vi "front_panel.vi"() -> ()   [LabVIEW 2020]
uses:
  kontolka.ctl
panel:
  out "unsigned 32bit integer":u32
  in  "Tab Control":enum32{"Page 1", "Page 2"}(tab)
  in  "Record Button":bool
  in  "Play Button":bool
  in  "Media Stop Button":bool
  out "Output panel":T1
  in  "Stop Button":bool
  in  "Control panel":T2
  in  "Open Button":bool
  in  "Save Button":bool
  in  "Configuration name":string
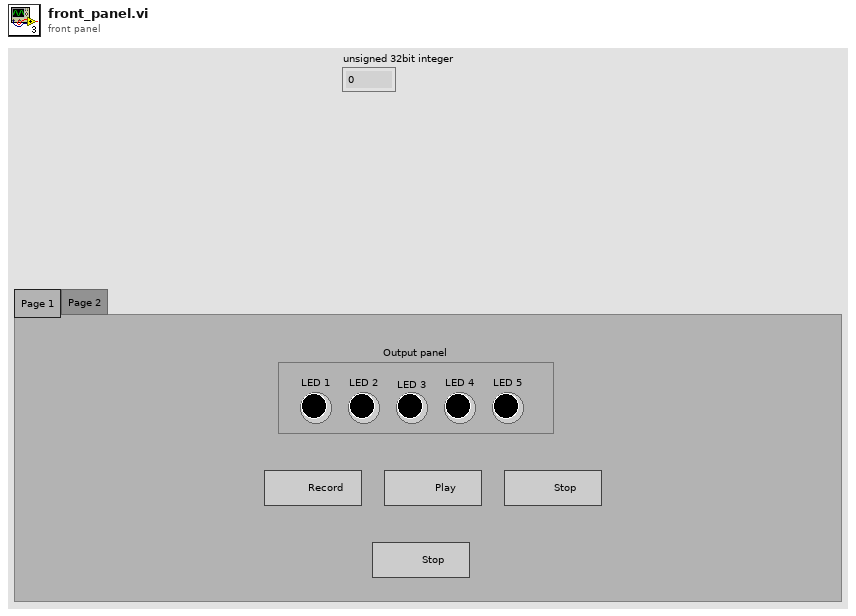
[diagram p1: front panel]
types:
  T1 = cluster{"LED 1":bool, "LED 2":bool, "LED 3":bool, "LED 4":bool, "LED 5":bool}
  T2 = cluster{"  LED 1":cluster{"Wait time":dbl, "Duration time":dbl, "Color":u32}, "  LED 2":cluster{"Wait time":dbl, "Duration time":dbl, "Color":u32}, "LED 3":cluster{"Wait time":dbl, "Duration time":dbl, "Color":u32}, "LED 4":cluster{"Wait time":dbl, "Duration time":dbl, "Color":u32}, " LED 5":cluster{"Wait time":dbl, "Duration time":dbl, "Color":u32}}
  T3 = typedef "kontolka.ctl" = enum16{"Init", "Record", "Play", "Stop", "Open", "Save", "PreparePlay"}
  T4 = enum32{"Page Enabled", "Page Disabled", "Page Disabled & Grayed"}
  T5 = cluster{"Wait time":dbl, "Duration time":dbl, u32}
  T6 = enum8{"Enabled", "Disabled", "Disabled and Grayed Out"}
  T7 = cluster{cluster{"String":i32, "String":i32, "String":i32}, cluster{"String":i32, "String":i32, "String":i32}, cluster{"String":i32, "String":i32, "String":i32}, cluster{"String":i32, "String":i32, "String":i32}, cluster{"String":i32, "String":i32, "String":i32}}
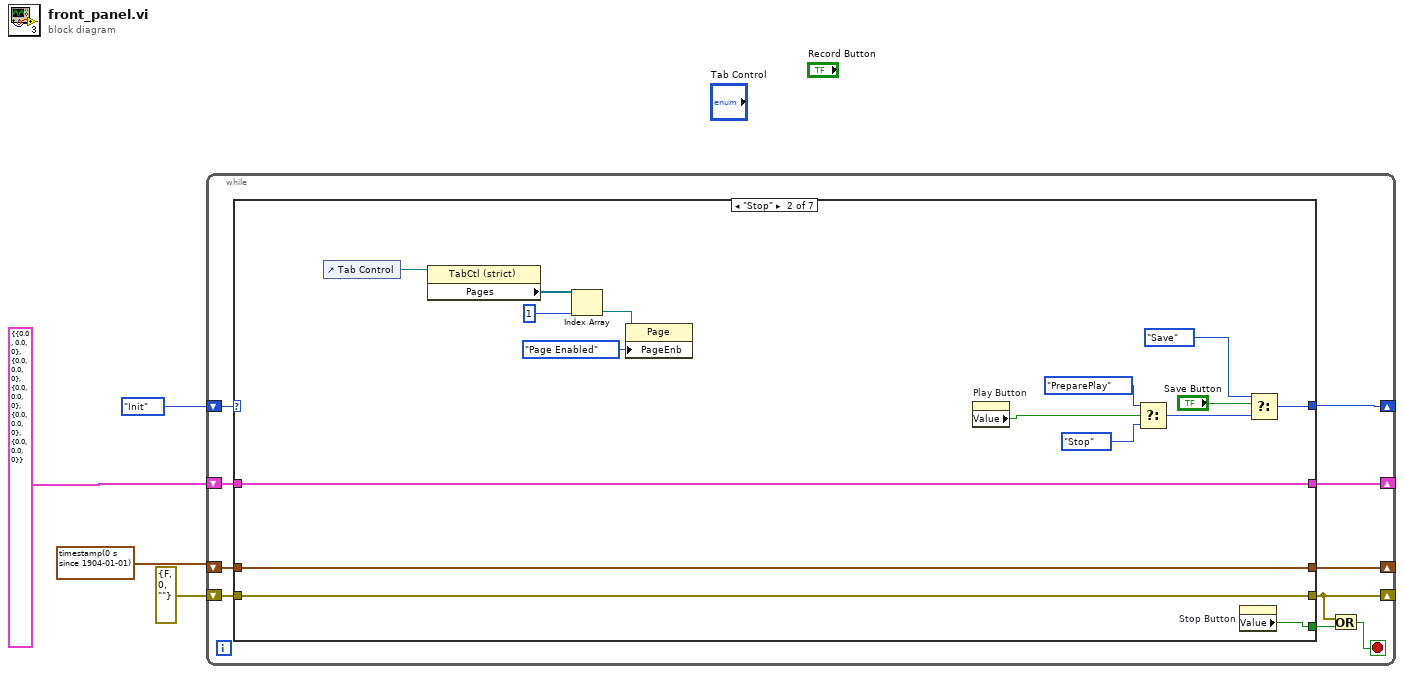
[diagram p0: block diagram]
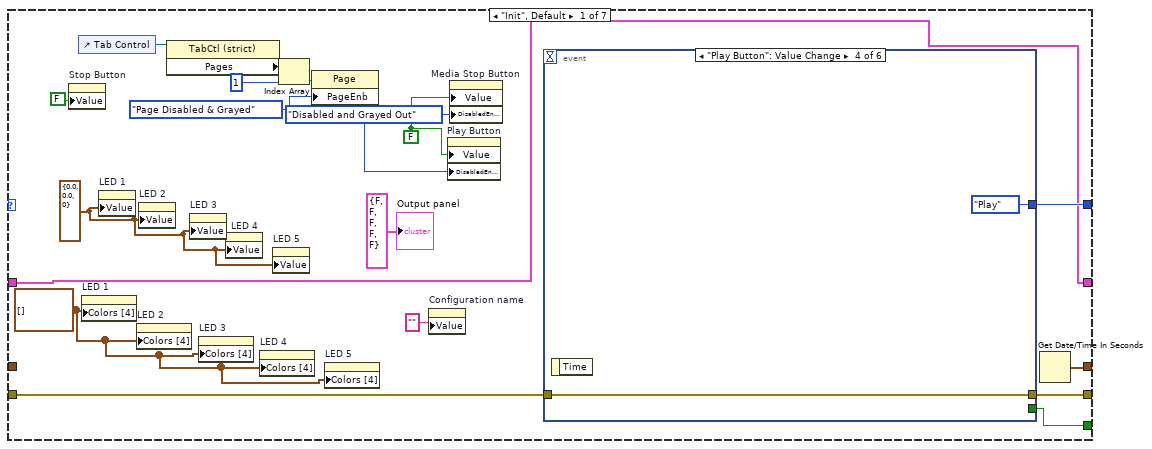
[diagram p2: hidden frame]
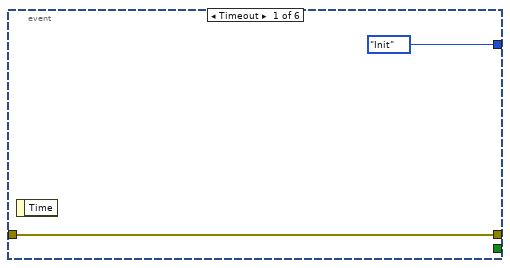
[diagram p3: hidden frame]
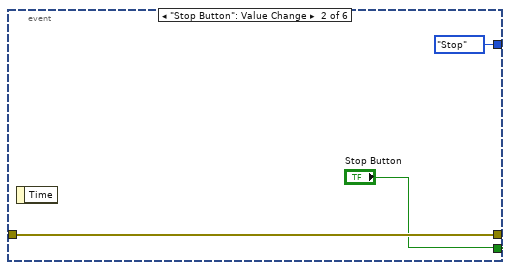
[diagram p4: hidden frame]
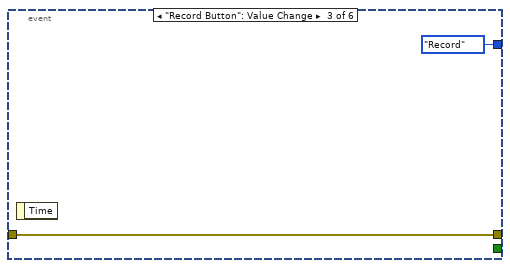
[diagram p5: hidden frame]
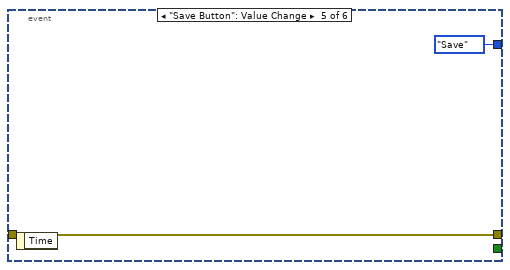
[diagram p6: hidden frame]
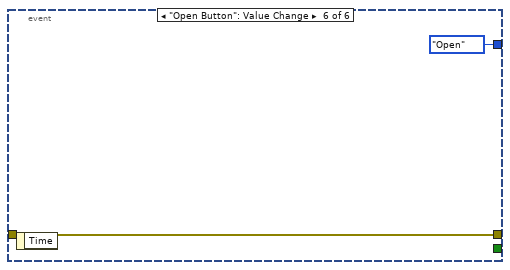
[diagram p7: hidden frame]
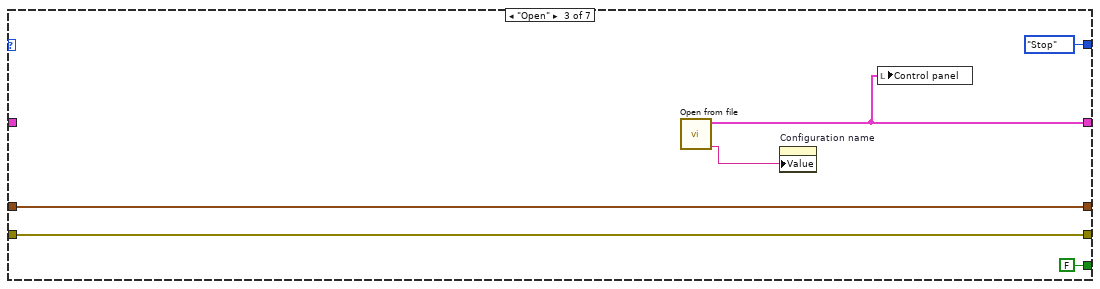
[diagram p8: hidden frame]
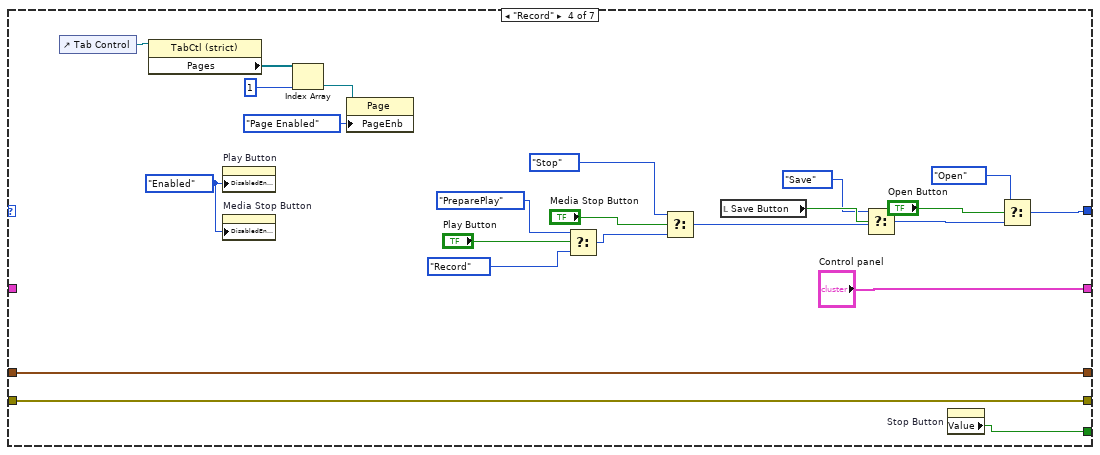
[diagram p9: hidden frame]
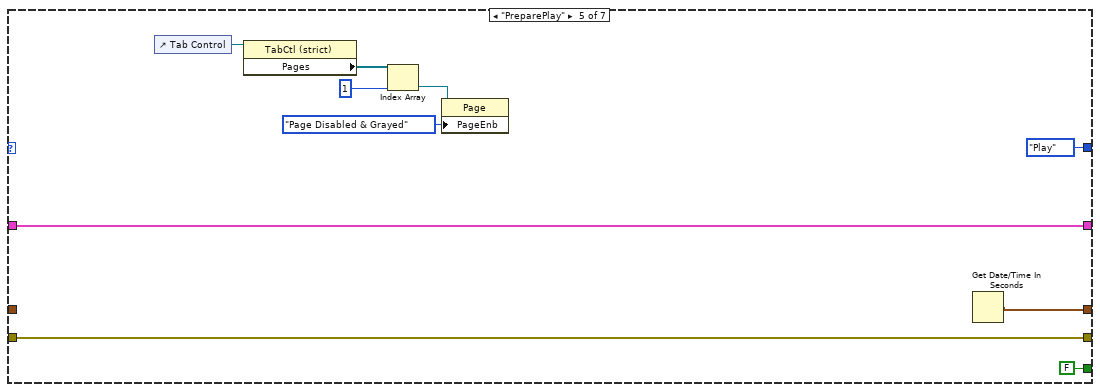
[diagram p10: hidden frame]
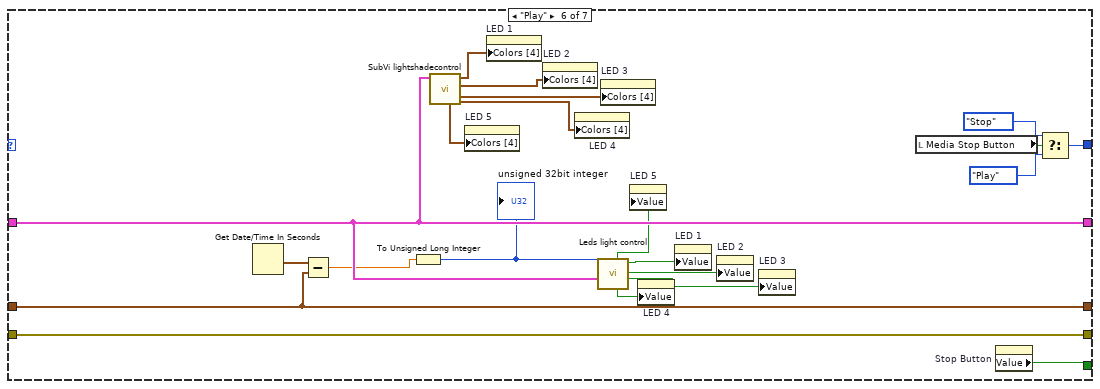
[diagram p11: hidden frame]
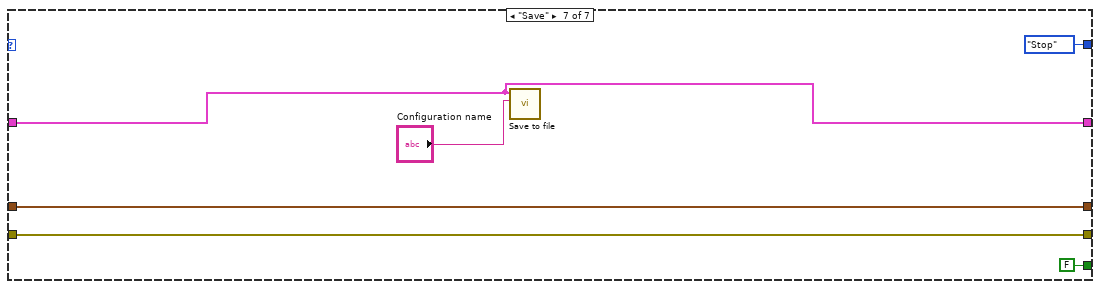
[diagram p12: hidden frame]
diagram:
  n1 = while {
    shift-right: [w11] -> _
    shift-left: errorcluster {"status"=FALSE, "code"=0, "source"=""} ("error constant") -> [w14]
    shift-right: [w5] -> _
    shift-left: kontolka."Init" ("Enum") -> [w10]
    shift-right: [w9] -> _
    shift-left: timestamp(0 s since 1904-01-01) ("seconds since 1Jan1904") -> [w8]
    shift-right: [w7] -> _
    shift-left: T2 {"  LED 1"={"Wait time"=0.0, "Duration time"=0.0, "Color"=0}, "  LED 2"={"Wait time"=0.0, "Duration time"=0.0, "Color"=0}, "LED 3"={"Wait time"=0.0, "Duration time"=0.0, "Color"=0}, "LED 4"={"Wait time"=0.0, "Duration time"=0.0, "Color"=0}, " LED 5"={"Wait time"=0.0, "Duration time"=0.0, "Color"=0}} ("Control panel") -> [w6]
    stop <- w12 stop-if-true
    n2 = case shown="\"Stop\"" w10 {
      tunnel: [w30 w60 w65 w90 w99 w121 w123] -> w11
      tunnel: w14 -> [w31 w60 w65 w90 w99 w121 w123]
      tunnel: [w29 w61 FALSE ("Value") w79 FALSE ("Value") w120 FALSE ("Value")] -> w13
      tunnel: [w32 w46 kontolka."Stop" ("Enum") w72 kontolka."Play" ("Enum") w119 kontolka."Stop" ("Enum")] -> w5
      tunnel: [w23 w59 w66 w78 w98 w108 w124] -> w9
      tunnel: w8 -> [_ w59 w66 w78 _ w108 w124]
      tunnel: [w21 w58 w62 "Control panel" w97 w110 w126] -> w7
      tunnel: w6 -> [w21 w58 _ _ w97 w110 w126]
      frame "Init", Default {
        w15 = cluster{u32, u32}[] [] ("Colors [4]")
        w17 = T5 {"Wait time"=0.0, "Duration time"=0.0, 0} ("Value")
        w19 = T6."Disabled and Grayed Out" ("Disabled")
        w20 = FALSE ("Media Stop Button")
        n3 = property on="Stop Button" class="Bool (strict)"("Value"=FALSE ("Stop Button")) -> ()  [unwired: 2 in, 2 out]
        n4 = control-ref of="Tab Control"() -> (w24:refnum<vi>)
        n5 = property on="LED 1" class="Bool (strict)"("Colors [4]"=w15) -> ()  [unwired: 2 in, 2 out]
        n6 = property on="LED 1" class="Clust (strict)"("Value"=w17) -> ()  [unwired: 2 in, 2 out]
        n7 = property on="LED 2" class="Bool (strict)"("Colors [4]"=w15) -> ()  [unwired: 2 in, 2 out]
        n8 = property on="LED 2" class="Clust (strict)"("Value"=w17) -> ()  [unwired: 2 in, 2 out]
        n9 = property on="Property Node" class="TabCtl (strict)"(reference=w24) -> ("Pages"=w27:refnum<vi>[])  [unwired: 1 in, 2 out]
        n10 = property on="LED 3" class="Clust (strict)"("Value"=w17) -> ()  [unwired: 2 in, 2 out]
        n11 = property on="LED 3" class="Bool (strict)"("Colors [4]"=w15) -> ()  [unwired: 2 in, 2 out]
        n12 = property on="LED 4" class="Clust (strict)"("Value"=w17) -> ()  [unwired: 2 in, 2 out]
        n13 = property on="LED 4" class="Bool (strict)"("Colors [4]"=w15) -> ()  [unwired: 2 in, 2 out]
        n14 = property on="LED 5" class="Clust (strict)"("Value"=w17) -> ()  [unwired: 2 in, 2 out]
        n15 = Index Array(array=w27, index=1) -> (element=w28:refnum<vi>)
        n16 = property class="Page"(reference=w28, "PageEnb"=T4."Page Disabled & Grayed" ("Page Enabled State")) -> ()  [unwired: 1 in, 2 out]
        n17 = property on="LED 5" class="Bool (strict)"("Colors [4]"=w15) -> ()  [unwired: 2 in, 2 out]
        n18 = property on="Configuration name" class="Str"("Value"="" ("Configuration name")) -> ()  [unwired: 2 in, 2 out]
        n19 = property on="Play Button" class="Bool (strict)"("Value"=w20, "DisabledEnum"=w19) -> ()  [unwired: 2 in, 2 out]
        n20 = property on="Media Stop Button" class="Bool (strict)"("Value"=w20, "DisabledEnum"=w19) -> ()  [unwired: 2 in, 2 out]
        n21 = event shown="[3] \"Play Button\": Value Change" {
          selector: _ -> [_ _ _ _ _ _]
          dyn-events: _ -> [_ _ _ _ _ _]
          timeout: _ -> [_ _ _ _ _ _]
          tunnel: [kontolka."Init" ("Enum") kontolka."Stop" ("Enum") kontolka."Record" ("Enum") kontolka."Play" ("Enum") kontolka."Save" ("Enum") kontolka."Open" ("Enum")] -> w32
          tunnel: w31 -> [w33 w37 w38 w41 w42 w44]
          tunnel: [w33 w37 w38 w41 w42 w44] -> w30
          tunnel: [_ "Stop Button" _ _ _ _] -> w29
          event Timeout {
            n22 = event-data() -> ()  [unwired: 1 in, 1 out]
          }
          event "Stop Button": Value Change {
            n23 = event-data() -> ()  [unwired: 1 in, 1 out]
          }
          event "Record Button": Value Change {
            n24 = event-data() -> ()  [unwired: 1 in, 1 out]
          }
          event "Play Button": Value Change {
            n25 = event-data() -> ()  [unwired: 1 in, 1 out]
          }
          event "Save Button": Value Change {
            n26 = event-data() -> ()  [unwired: 1 in, 1 out]
          }
          event "Open Button": Value Change {
            n27 = event-data() -> ()  [unwired: 1 in, 1 out]
          }
        }
        n28 = Get Date/Time In Seconds() -> (seconds since 1Jan1904=w23:timestamp)
        "Output panel" <- T1 {"LED 1"=FALSE, "LED 2"=FALSE, "LED 3"=FALSE, "LED 4"=FALSE, "LED 5"=FALSE} ("Output panel")
      }
      frame "Stop" {
        n29 = control-ref of="Tab Control"() -> (w50:refnum<vi>)
        n30 = property on="Property Node" class="TabCtl (strict)"(reference=w50) -> ("Pages"=w54:refnum<vi>[])  [unwired: 1 in, 2 out]
        n31 = Index Array(array=w54, index=1) -> (element=w53:refnum<vi>)
        n32 = property class="Page"(reference=w53, "PageEnb"=T4."Page Enabled" ("Page Enabled State")) -> ()  [unwired: 1 in, 2 out]
        n33 = property on="Play Button" class="Bool (strict)"() -> ("Value"=w57:bool)  [unwired: 2 in, 2 out]
        n34 = Select(t=kontolka."PreparePlay" ("Enum"), s=w57, f=kontolka."Stop" ("Enum")) -> (s? t:f=w49:T3)
        n35 = property on="Stop Button" class="Bool (strict)"() -> ("Value"=w61:bool)  [unwired: 2 in, 2 out]
        n36 = Select(t=kontolka."Save", s="Save Button", f=w49) -> (s? t:f=w46:T3)
      }
      frame "Open" {
        n37 = call "Open from file.vi"() -> ("Confign name"=w63:string, "Cluster"=w62:T7)  [unwired: 10 in]
        n38 = property on="Configuration name" class="Str"("Value"=w63) -> ()  [unwired: 2 in, 2 out]
        n39 = local write "Control panel"(w62) -> ()
      }
      frame "Record" {
        w76 = T6."Enabled" ("Disabled")
        n40 = control-ref of="Tab Control"() -> (w86:refnum<vi>)
        n41 = property on="Property Node" class="TabCtl (strict)"(reference=w86) -> ("Pages"=w89:refnum<vi>[])  [unwired: 1 in, 2 out]
        n42 = property on="Play Button" class="Bool (strict)"("DisabledEnum"=w76) -> ()  [unwired: 2 in, 2 out]
        n43 = property on="Media Stop Button" class="Bool (strict)"("DisabledEnum"=w76) -> ()  [unwired: 2 in, 2 out]
        n44 = Index Array(array=w89, index=1) -> (element=w88:refnum<vi>)
        n45 = property class="Page"(reference=w88, "PageEnb"=T4."Page Enabled" ("Page Enabled State")) -> ()  [unwired: 1 in, 2 out]
        n46 = Select(t=kontolka."PreparePlay" ("Enum"), s="Play Button", f=kontolka."Record" ("Enum")) -> (s? t:f=w82:T3)
        n47 = Select(t=kontolka."Stop" ("Enum"), s="Media Stop Button", f=w82) -> (s? t:f=w74:T3)
        n48 = local read "Save Button"() -> (w70:bool)
        n49 = Select(t=kontolka."Save", s=w70, f=w74) -> (s? t:f=w73:T3)
        n50 = property on="Stop Button" class="Bool (strict)"() -> ("Value"=w79:bool)  [unwired: 2 in, 2 out]
        n51 = Select(t=kontolka."Open", s="Open Button", f=w73) -> (s? t:f=w72:T3)
      }
      frame "PreparePlay" {
        n52 = control-ref of="Tab Control"() -> (w92:refnum<vi>)
        n53 = property on="Property Node" class="TabCtl (strict)"(reference=w92) -> ("Pages"=w95:refnum<vi>[])  [unwired: 1 in, 2 out]
        n54 = Index Array(array=w95, index=1) -> (element=w96:refnum<vi>)
        n55 = property class="Page"(reference=w96, "PageEnb"=T4."Page Disabled & Grayed" ("Page Enabled State")) -> ()  [unwired: 1 in, 2 out]
        n56 = Get Date/Time In Seconds() -> (seconds since 1Jan1904=w98:timestamp)
      }
      frame "Play" {
        n57 = Get Date/Time In Seconds() -> (seconds since 1Jan1904=w109:timestamp)
        n58 = Subtract(x=w109, y=w108) -> (x-y=w107:dbl)
        n59 = To Unsigned Long Integer(number=w107) -> (unsigned 32bit integer=w106:u32)
        "unsigned 32bit integer" <- w106
        n60 = call "SubVi lightshadecontrol.vi"("Control panel"=w110) -> ("LED 4"=w112:cluster{"Color":u32, "Color":u32}[], "LED 3"=w113:cluster{"Color":u32, "Color":u32}[], "LED 2"=w114:cluster{"Color":u32, "Color":u32}[], "LED 1"=w115:cluster{"Color":u32, "Color":u32}[], "LED 5"=w111:cluster{"Color":u32, "Color":u32}[])  [unwired: 6 in]
        n61 = property on="LED 5" class="Bool (strict)"("Colors [4]"=w111) -> ()  [unwired: 2 in, 2 out]
        n62 = property on="LED 1" class="Bool (strict)"("Colors [4]"=w115) -> ()  [unwired: 2 in, 2 out]
        n63 = property on="LED 2" class="Bool (strict)"("Colors [4]"=w114) -> ()  [unwired: 2 in, 2 out]
        n64 = property on="LED 4" class="Bool (strict)"("Colors [4]"=w112) -> ()  [unwired: 2 in, 2 out]
        n65 = call "Leds light control.vi"("Control panel"=w110, "number"=w106) -> ("LED 3"=w103:bool, "LED 2"=w104:bool, "LED 1"=w105:bool, "LED 4"=w102:bool, "LED 5"=w101:bool)  [unwired: 5 in]
        n66 = property on="LED 3" class="Bool (strict)"("Colors [4]"=w113) -> ()  [unwired: 2 in, 2 out]
        n67 = property on="LED 5" class="Bool (strict)"("Value"=w101) -> ()  [unwired: 2 in, 2 out]
        n68 = property on="LED 4" class="Bool (strict)"("Value"=w102) -> ()  [unwired: 2 in, 2 out]
        n69 = property on="LED 1" class="Bool (strict)"("Value"=w105) -> ()  [unwired: 2 in, 2 out]
        n70 = property on="LED 2" class="Bool (strict)"("Value"=w104) -> ()  [unwired: 2 in, 2 out]
        n71 = property on="LED 3" class="Bool (strict)"("Value"=w103) -> ()  [unwired: 2 in, 2 out]
        n72 = local read "Media Stop Button"() -> (w118:bool)
        n73 = property on="Stop Button" class="Bool (strict)"() -> ("Value"=w120:bool)  [unwired: 2 in, 2 out]
        n74 = Select(t=kontolka."Stop" ("Enum"), s=w118, f=kontolka."Play" ("Enum")) -> (s? t:f=w119:T3)
      }
      frame "Save" {
        n75 = call "Save to file.vi"("String"="Configuration name", "Control panel"=w126) -> ()  [unwired: 10 in]
      }
    }
    n76 = Or(x=w11, y=w13) -> (x .or. y?=w12:bool)
  }
